vi "Global 1.vi"() -> ()   [LabVIEW 2024]
panel:
  in  "D":dbl
  in  "C":dbl
  in  "B":bool
  in  "A":bool
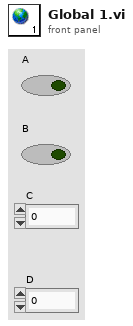
[diagram p1: front panel]
diagram:
